vi "SRV_Append Array of Strings with Separators.vi"(0 "Initial String":string, 7 "Array of Strings to Append":string[](array[string]), 9 "Element Separator(, )":string=", ", 11 "Trim Output String (T)":bool=TRUE) -> (8 "String Out":string)   [LabVIEW 2014]
doc: "Appends an array of strings to an initial string. The elements of the array are separated by the Element Separator string.\n\nAuthor: Mike Schultz"
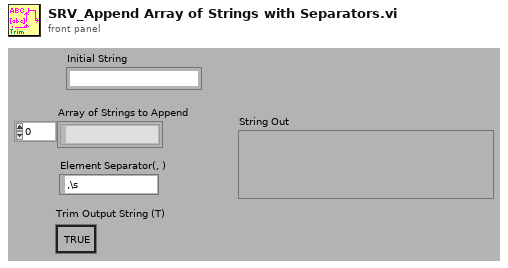
[diagram p1: front panel]
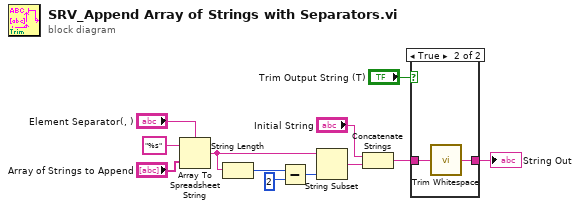
[diagram p0: block diagram]
diagram:
  n1 = Array To Spreadsheet String(delimiter (Tab)="Element Separator(, )", array="Array of Strings to Append", 3:"%s" ("format string")) -> (spreadsheet string=w2:string)
  n2 = String Length(string=w2) -> (length=w5:i32)
  n3 = Subtract(x=w5, y=2) -> (x-y=w3:i32)
  n4 = String Subset(string=w2, length (rest)=w3) -> (substring=w1:string)  [unwired: 1 out]
  n5 = Concatenate Strings("Initial String", w1) -> (w8:string)
  n6 = case shown="True" "Trim Output String (T)" {
    tunnel: [w13 w15] -> w6
    tunnel: w8 -> [w13 w14]
    frame False {
    }
    frame True {
      n7 = call <vilib>:"Trim Whitespace.vi"("string"=w14) -> ("trimmed string"=w15:string)  [unwired: 1 in]
    }
  }
  "String Out" <- w6
